vi "updateCANtable.vi"(8 "error in (no error)":errorcluster, 11 "CANtable.in":refnum<class "bAPPdata.lvclass">) -> (0 "error out":errorcluster, 3 "CANtable.out":refnum<class "bAPPdata.lvclass">)   [LabVIEW 2015, in "bAPPdata.lvclass"]
doc: "This VI converts the data returned by ncReadNetMult into a two-dimensional array of strings."
uses:
  bAPPdata.lvclass
  bAPPdata.lvclass/bAPPdata.ctl
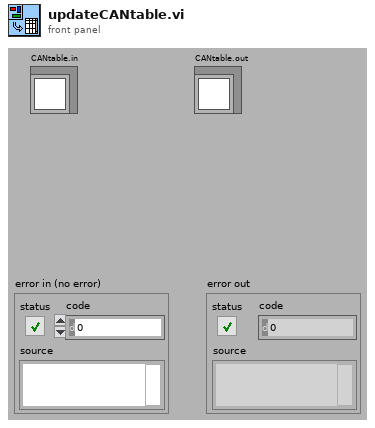
[diagram p1: front panel]
types:
  T1 = typedef "bAPPdata.lvclass/table-data.ctl" = T2[]
  T2 = typedef "bAPPdata.lvclass/table-contents.ctl" = cluster{"id":u32, "tag":string, "frame.type":T3, "last.frame":T4, "tMsgData":T6, "child.tags":string[], "bit-payload":bool[]}
  T3 = typedef "frame.type.ctl" = enum16{"FRAME NOT DEFINED", "DUT OUTPUT FRAME", "DUT INPUT FRAME"}
  T4 = typedef "XNET Frame CAN.ctl" = cluster{"timestamp":timestamp, "payload":u8[], "identifier":u32, "type":T5, "extended?":bool, "echo?":bool}
  T5 = typedef "XNET Frame Type CAN.ctl" = u8
  T6 = typedef "nMsgData.ctl" = cluster{"dwID":u32, "count":u32, "dwCycleTime":dbl, "dwTime":dbl, "new msg":bool}
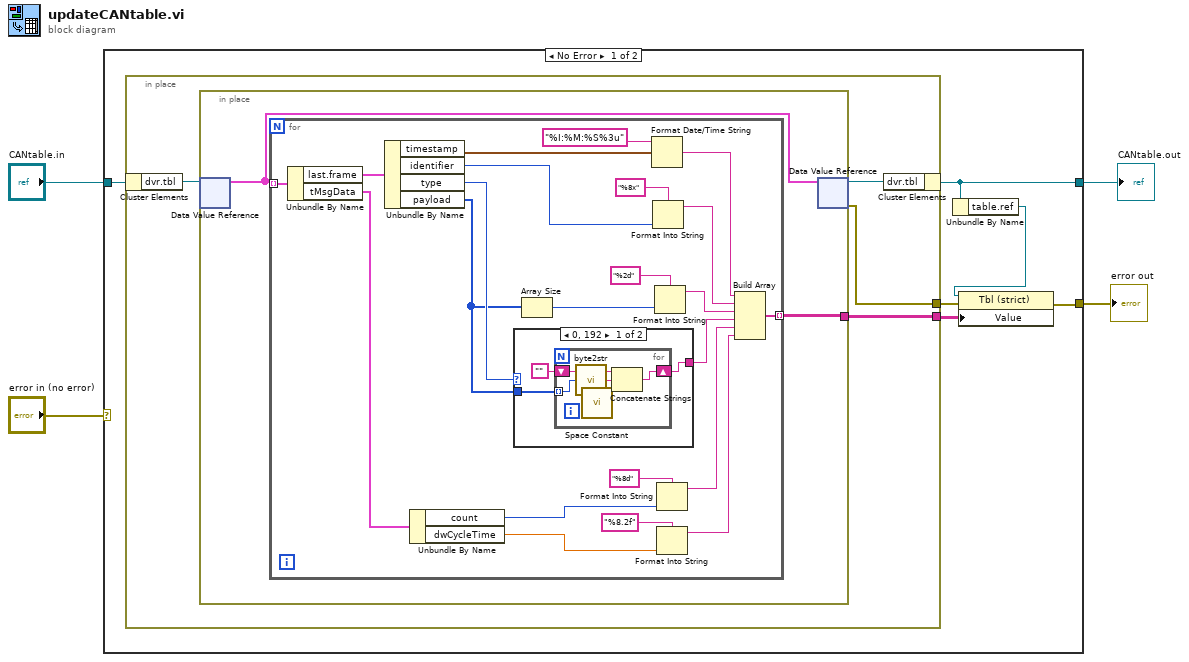
[diagram p0: block diagram]
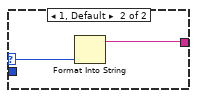
[diagram p2: hidden frame]
diagram:
  n1 = case shown="No Error" "error in (no error)" {
    selector: "error in (no error)" -> [_ w50]
    tunnel: [w9 w50] -> w3
    tunnel: "CANtable.in" -> [w7 w49]
    tunnel: [w6 w49] -> w1
    frame No Error {
      n2 = in-place {
        in-place-border: [w13] -> w10
        in-place-border: [w11] -> w8
        n3 = in-place-cluster #1(w7) -> ("dvr.tbl"=w14:refnum<data-value>)
        n4 = in-place {
          in-place-border: [w16] -> w11
          n5 = in-place-dvr #2(w14) -> (w15:T1)  [unwired: 1 out]
          n6 = for {
            tunnel: [w29] -> w16 mode=indexing
            tunnel: w15 -> [w17] mode=indexing
            n7 = Unbundle By Name(w17) -> ("last.frame"=w24:T4, "tMsgData"=w25:T6)
            n8 = Unbundle By Name(w24) -> ("timestamp"=w27:timestamp, "identifier"=w37:u32, "type"=w23:T5, "payload"=w19:u8[])
            n9 = Unbundle By Name(w25) -> ("count"=w33:u32, "dwCycleTime"=w31:dbl)
            n10 = case shown="0, 192" w23 {
              selector: w23 -> [_ w48]
              tunnel: [w39 w47] -> w22
              tunnel: w19 -> [w41 _]
              frame 0, 192 {
                n11 = for {
                  tunnel: w41 -> [w42] mode=indexing
                  shift-right: [w45] -> w39
                  shift-left: "" -> [w46]
                  n12 = call "byte2str.vi"("byte"=w42) -> ("String"=w43:string)  [unwired: 4 in]
                  n13 = call <vilib>:"Space Constant.vi"() -> ("String"=w44:string)
                  n14 = Concatenate Strings(w46, w43, w44) -> (w45:string)
                }
              }
              frame 1, Default {
                n15 = Format Into String(w48) -> (resulting string=w47:string)  [unwired: 3 in, 1 out]
              }
            }
            n16 = Array Size(array=w19) -> (size(s)=w18:i32)
            n17 = Format Date/Time String(time format string (%c)="%I:%M:%S%3u", seconds (now)=w27) -> (date/time string=w26:string)  [unwired: 1 out]
            n18 = Format Into String(format string="%8x", w37) -> (resulting string=w36:string)  [unwired: 2 in, 1 out]
            n19 = Format Into String(format string="%2d" ("Format String"), w18) -> (resulting string=w35:string)  [unwired: 2 in, 1 out]
            n20 = Format Into String(format string="%8d", w33) -> (resulting string=w32:string)  [unwired: 2 in, 1 out]
            n21 = Format Into String(format string="%8.2f", w31) -> (resulting string=w21:string)  [unwired: 2 in, 1 out]
            n22 = Build Array(w26, w36, w35, w22, w32, w21) -> (w29:string[])
          }
          n23 = in-place-dvr #2(w15) -> (w12:refnum<data-value>, w13:errorcluster)
        }
        n24 = in-place-cluster #1("dvr.tbl"=w12) -> (w6:refnum<class "bAPPdata.lvclass">)
      }
      n25 = Unbundle By Name(w6) -> ("table.ref"=w5:refnum<vi>)
      n26 = property class="Tbl (strict)"(reference=w5, error in=w10, "Value"=w8) -> (error out=w9:errorcluster)  [unwired: 1 out]
    }
    frame Error {
    }
  }
  "CANtable.out" <- w1
  "error out" <- w3
